vi "Split into 2.vi"(0 "Cx":dbl[](array[numeric]), 5 "Cy":dbl[](array[numeric]), 7 "Ix":dbl[](array[numeric]), 9 "Iy":dbl[](array[numeric]), 11 "X":u8[](array[numeric])) -> (2 "C1x":dbl[](array[numeric]), 3 "C1y":dbl[](array[numeric]), 4 "C2x":dbl[](array[numeric]), 6 "C2y":dbl[](array[numeric]))   [LabVIEW 2023, in "d15.lvlib" / "Cave.lvclass"]
uses:
  Cave.lvclass
  Diamond/Diamond.lvclass
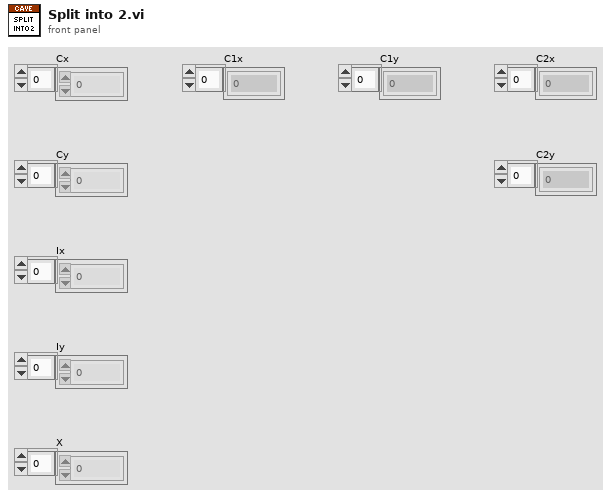
[diagram p1: front panel]
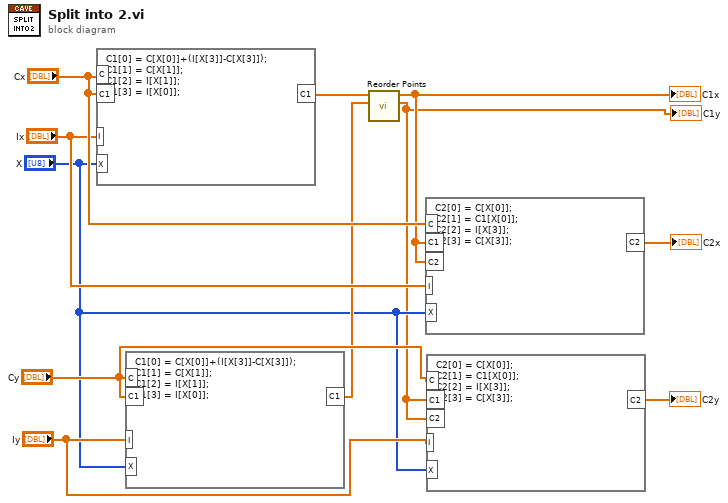
[diagram p0: block diagram]
diagram:
  n1 = formula code="C1[0] = C[X[0]]+(I[X[3]]-C[X[3]]);\nC1[1] = C[X[1]];\nC1[2] = I[X[1]];\nC1[3] = I[X[0]];"("C"="Cx", "I"="Ix", "X"="X", "C1"="Cx") -> ("C1"=w11:dbl[])
  n2 = formula code="C1[0] = C[X[0]]+(I[X[3]]-C[X[3]]);\nC1[1] = C[X[1]];\nC1[2] = I[X[1]];\nC1[3] = I[X[0]];"("C"="Cy", "I"="Iy", "X"="X", "C1"="Cy") -> ("C1"=w7:dbl[])
  n3 = call "Reorder Points.vi"("Y"=w7, "X"=w11) -> ("Y'"=w3:dbl[], "X'"=w4:dbl[])  [unwired: 8 in]
  "C1x" <- w4
  "C1y" <- w3
  n4 = formula code="C2[0] = C[X[0]];\nC2[1] = C1[X[0]];\nC2[2] = I[X[3]];\nC2[3] = C[X[3]];"("C"="Cx", "I"="Ix", "X"="X", "C1"=w4, "C2"=w4) -> ("C2"=→"C2x":dbl[])
  n5 = formula code="C2[0] = C[X[0]];\nC2[1] = C1[X[0]];\nC2[2] = I[X[3]];\nC2[3] = C[X[3]];"("C"="Cy", "I"="Iy", "X"="X", "C1"=w3, "C2"=w3) -> ("C2"=→"C2y":dbl[])
